vi "Clean Error Source String.vi"(11 "Error Source String":string) -> (3 "Cleaned Error String":string)   [LabVIEW 2016, in "hse-logger.lvlib" / "Formatter.lvclass"]
uses:
  Formatter.lvclass
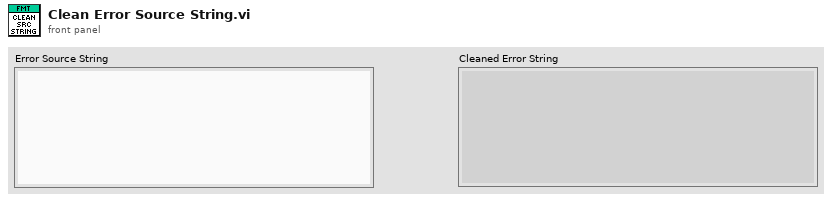
[diagram p1: front panel]
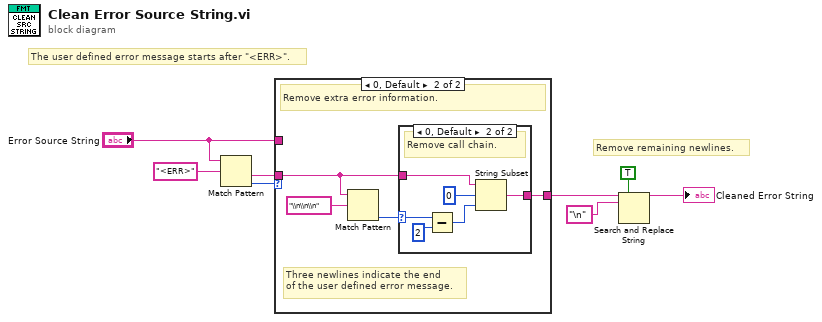
[diagram p0: block diagram]
diagram:
  # "Remove remaining newlines."
  # "The user defined error message starts after \"<ERR>\"."
  n1 = Match Pattern(string="Error Source String", regular expression="<ERR>") -> (after substring=w7:string, offset past match=w2:i32)  [unwired: 1 in, 2 out]
  n2 = case shown="0, Default" w2 {
    tunnel: w7 -> [_ w11]
    tunnel: [w9 w10] -> w6
    tunnel: "Error Source String" -> [w9 _]
    frame -1 {
      # "No \"<ERR>\" tag in string."
    }
    frame 0, Default {
      # "Three newlines indicate the end\nof the user defined error message."
      # "Remove extra error information."
      n3 = Match Pattern(string=w11, regular expression="\\n\\n\\n") -> (offset past match=w12:i32)  [unwired: 1 in, 3 out]
      n4 = case shown="0, Default" w12 {
        selector: w12 -> [_ w17]
        tunnel: w11 -> [w14 w16]
        tunnel: [w14 w15] -> w10
        frame -1 {
          # "No call chain."
        }
        frame 0, Default {
          # "Remove call chain."
          n5 = Subtract(x=w17, y=2 ("x")) -> (x-y=w19:i32)
          n6 = String Subset(string=w16, offset (0)=0, length (rest)=w19) -> (substring=w15:string)
        }
      }
    }
  }
  n7 = Search and Replace String(replace all?=TRUE ("replace all? (F)"), input string=w6, search string="\n") -> (result string=→"Cleaned Error String":string)  [unwired: 5 in, 3 out]
